vi "accelero_et_led.vi"() -> ()   [LabVIEW 2019]
uses:
  <vilib>/myRIO/Express VI/Onboard Devices/Accelerometer/Accelerometer Express VI.xnode
  <vilib>/myRIO/Instrument Drivers/Onboard Devices/Accelerometer/typedefs/Accelerometer Reference.ctl
  <vilib>/myRIO/Instrument Drivers/Onboard Devices/Accelerometer/Accelerometer.lvlib
  <vilib>/myRIO/Common/Instrument Driver Framework/myRIO v1.0/Accelerometer/typedefs/Accelerometer Channels List.ctl
  <vilib>/myRIO/Common/Instrument Driver Framework/myRIO v1.0/Accelerometer/typedefs/Accelerometer Channels Enum.ctl
  <vilib>/myRIO/Common/Instrument Driver Framework/Utilities/typedefs/myRIO Generic Hardware Reference.ctl
  <vilib>/myRIO/Common/Instrument Driver Framework/Utilities/typedefs/myRIO v1.0 Reference.ctl
  <vilib>/myRIO/Common/Instrument Driver Framework/Utilities/typedefs/Generic FPGA Reference.ctl
  <vilib>/myRIO/Common/Instrument Driver Framework/Utilities/typedefs/Hardware Version Enum.ctl
  <vilib>/myRIO/Instrument Drivers/Onboard Devices/Accelerometer/vis/Read.vi
  <vilib>/myRIO/Instrument Drivers/Onboard Devices/Accelerometer/vis/myRIO Accelerometer Open.xnode
  <vilib>/userDefined/High Color/nirio_resource_hc.ctl
  <vilib>/myRIO/Common/Instrument Driver Framework/Utilities/vis/Is FPGA Ref Available.vi
  <vilib>/myRIO/Common/Instrument Driver Framework/myRIO v1.0/DIO/typedefs/DIO Channels Enum.ctl
  <vilib>/myRIO/Common/Instrument Driver Framework/myRIO v1.0/DIO/typedefs/DIO Channels List.ctl
  <vilib>/myRIO/Instrument Drivers/Onboard IO/DIO/typedefs/DIO Reference.ctl
  <vilib>/myRIO/Instrument Drivers/Onboard IO/DIO/DIO.lvlib
  <vilib>/myRIO/Instrument Drivers/Onboard IO/DIO/vis/myRIO DIO Open.xnode
  <vilib>/myRIO/Common/Instrument Driver Framework/myRIO v1.0/DIO/vis/myRIO v1.1 Open DIO.vi
  <vilib>/myRIO/Express VI/Onboard IO/DI/DI Express VI.xnode
  <vilib>/myRIO/Instrument Drivers/Onboard IO/DIO/vis/Read.vi
  <vilib>/myRIO/Express VI/Onboard Devices/LED/LED Express VI.xnode
  <vilib>/myRIO/Instrument Drivers/Onboard IO/DIO/vis/Write.vi
  <vilib>/myRIO/Common/Instrument Driver Framework/myRIO v1.0/Accelerometer/vis/myRIO v1.1 Open Accelerometer.vi
panel:
  out "X 5":dbl(graph)
  out "X 4":dbl(graph)
  out "X 3":dbl(graph)
  out "X 2":dbl(graph)
  out "X":dbl(graph)
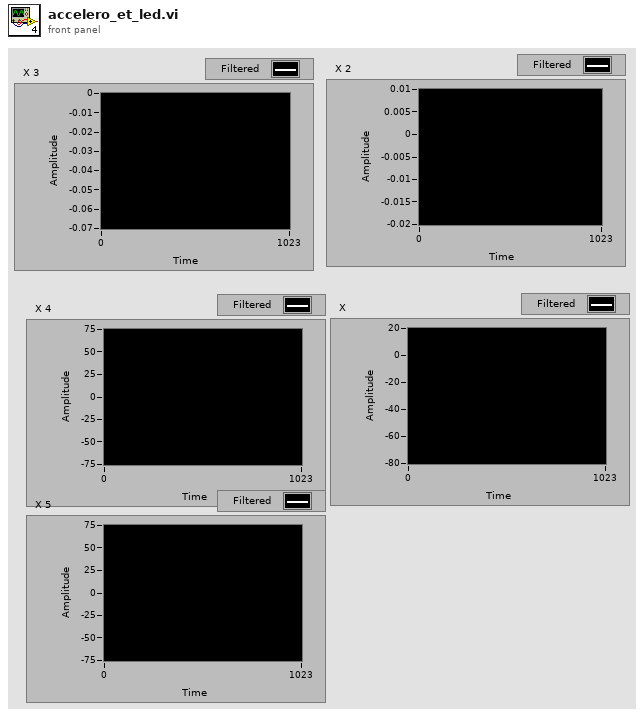
[diagram p1: front panel]
types:
  T1 = typedef "DIO.lvlib/DIO Reference.ctl" = cluster{"myRIO Reference":T2, "DIO Channels List":T6}
  T2 = typedef "myRIO Generic Hardware Reference.ctl" = cluster{"myRIO Model":T3, "myRIO Hardware Reference":T4}
  T3 = typedef "Hardware Version Enum.ctl" = enum16{"Unknown", "myRIO-1900", "myRIO-1950", "roboRIO", "NI ELVIS RIO CM", "ELVIS III"}
  T4 = typedef "myRIO v1.0 Reference.ctl" = cluster{"Generic FPGA Reference":T5, "Allow multiple opens":bool}
  T5 = typedef "Generic FPGA Reference.ctl" = refnum<k20>
  T6 = typedef "DIO Channels List.ctl" = T7[]
  T7 = typedef "DIO Channels Enum.ctl" = enum16{"Not Connected", "C/DIO0", "C/DIO1", "C/DIO2", "C/DIO3", "C/DIO4", "C/DIO5", "C/DIO6", "C/DIO7", "A/DIO0", "A/DIO1", "A/DIO2", "A/DIO3", "A/DIO4", "A/DIO5", "A/DIO6", "A/DIO7", "A/DIO8", "A/DIO9", "A/DIO10", "A/DIO11", "A/DIO12", "A/DIO13", "A/DIO14", "A/DIO15", "A/DIO16", "A/DIO17", "A/DIO18", "A/DIO19", "B/DIO0", "B/DIO1", "B/DIO2", "B/DIO3", "B/DIO4", "B/DIO5", "B/DIO6", "B/DIO7", "B/DIO8", "B/DIO9", "B/DIO10", "B/DIO11", "B/DIO12", "B/DIO13", "B/DIO14", "B/DIO15", "B/DIO16", "B/DIO17", "B/DIO18", "B/DIO19", "LED0", "LED1", "LED2", "LED3", "Button0", "DIO/DIO0", "DIO/DIO1", "DIO/DIO2", "DIO/DIO3", "DIO/DIO4", "DIO/DIO5", "DIO/DIO6", "DIO/DIO7", "DIO/DIO8", "DIO/DIO9", "SPI/CS0", "SPI/CS1", "SPI/CS2", "SPI/CS3", "LED RADIO (Green)", "LED RADIO (Red)", "LED COMM (Green)", "LED COMM (Red)", "LED MODE (Green)", "LED MODE (Red)"}
  T8 = typedef "nirio_resource_hc.ctl" = tag
  T9 = typedef "Accelerometer.lvlib/Accelerometer Reference.ctl" = cluster{"myRIO Reference":T2, "Accelerometer Channels List":T10, "LSB Weight":dbl}
  T10 = typedef "Accelerometer Channels List.ctl" = T11[]
  T11 = typedef "Accelerometer Channels Enum.ctl" = enum16{"Not Connected", "X-Axis", "Y-Axis", "Z-Axis"}
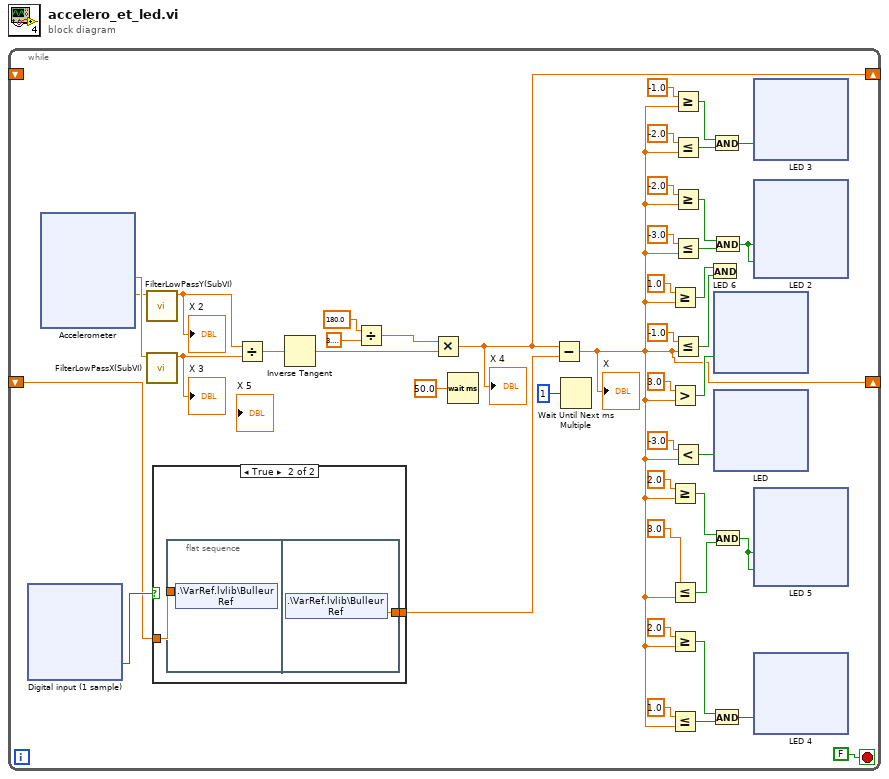
[diagram p0: block diagram]
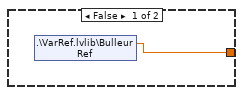
[diagram p2: hidden frame]
diagram:
  n1 = while {
    shift-right: [w5] -> _
    shift-left: _ -> [_]
    shift-right: [w4] -> _
    shift-left: _ -> [w2]
    stop <- FALSE stop-if-true
    n2 = xnode "Digital input (1 sample)"() -> ("A/DIO0 (Pin 11)"=w3:bool)  [unwired: 1 in, 1 out]
    n3 = xnode "Accelerometer"() -> ("X-Axis"=w9:dbl, "Y-Axis"=w8:dbl)  [unwired: 1 in, 2 out]
    n4 = call "FilterLowPassY(SubVI).vi"("Y-Axis"=w8) -> ("Filtered x"=w6:dbl)  [unwired: 9 in, 1 out]
    "X 2" <- w6
    n5 = call "FilterLowPassX(SubVI).vi"("X-Axis"=w9) -> ("Filtered x"=w7:dbl)  [unwired: 9 in, 1 out]
    "X 3" <- w7
    n6 = case shown="True" w3 {
      tunnel: w2 -> [_ w83]
      tunnel: [w81 w82] -> w1
      frame False {
        n7 = shared-variable ".\\VarRef.lvlib\\Bulleur Ref"() -> (w81:dbl)  [unwired: 1 in, 1 out]
      }
      frame True {
        n8 = flat-sequence {
          tunnel: w83 -> [w84]
          tunnel: [w85] -> w82
          frame #0 {
            n9 = shared-variable ".\\VarRef.lvlib\\Bulleur Ref"(w84) -> ()  [unwired: 1 in, 1 out]
          }
          frame #1 {
            n10 = shared-variable ".\\VarRef.lvlib\\Bulleur Ref"() -> (w85:dbl)  [unwired: 1 in, 1 out]
          }
        }
      }
    }
    n11 = Divide(x=w6, y=w7) -> (x/y=w44:dbl)
    n12 = Inverse Tangent(1:w44) -> (0:w43:dbl)
    n13 = Divide(x=180.0, y=3.141592653589793) -> (x/y=w40:dbl)
    n14 = Multiply(x=w40, y=w43) -> (x*y=w5:dbl)
    "X 4" <- w5
    n15 = Wait (ms)(milliseconds to wait=50.0) -> ()  [unwired: 1 out]
    n16 = Subtract(x=w5, y=w1) -> (x-y=w4:dbl)
    "X" <- w4
    n17 = Wait Until Next ms Multiple(millisecond multiple=1) -> ()  [unwired: 1 out]
    n18 = Greater Or Equal?(x=1.0, y=w4) -> (x >= y?=w27:bool)
    n19 = Greater?(x=3.0, y=w4) -> (0:w11:bool)
    n20 = Greater Or Equal?(x=2.0, y=w4) -> (x >= y?=w35:bool)
    n21 = Less Or Equal?(x=3.0, y=w4) -> (x <= y?=w33:bool)
    n22 = Greater Or Equal?(x=2.0, y=w4) -> (x >= y?=w31:bool)
    n23 = Less Or Equal?(x=1.0, y=w4) -> (x <= y?=w30:bool)
    n24 = Greater Or Equal?(x=-1.0, y=w4) -> (x >= y?=w23:bool)
    n25 = Less Or Equal?(x=-2.0, y=w4) -> (x <= y?=w22:bool)
    n26 = Greater Or Equal?(x=-2.0, y=w4) -> (x >= y?=w19:bool)
    n27 = Less Or Equal?(x=-3.0, y=w4) -> (x <= y?=w17:bool)
    n28 = Less Or Equal?(x=-1.0, y=w4) -> (x <= y?=w26:bool)
    n29 = Less?(x=-3.0, y=w4) -> (x < y?=w16:bool)
    n30 = And(x=w27, y=w26) -> ()  [unwired: 1 out]
    n31 = And(x=w23, y=w22) -> (x .and. y?=w14:bool)
    n32 = And(x=w31, y=w30) -> (x .and. y?=w13:bool)
    n33 = And(x=w19, y=w17) -> (x .and. y?=w15:bool)
    n34 = And(x=w35, y=w33) -> (x .and. y?=w12:bool)
    n35 = xnode "LED 6"("LED3"=w11) -> ()  [unwired: 1 in, 1 out]
    n36 = xnode "LED"("LED0"=w16) -> ()  [unwired: 1 in, 1 out]
    n37 = xnode "LED 3"("LED1"=w14) -> ()  [unwired: 1 in, 1 out]
    n38 = xnode "LED 2"("LED0"=w15, "LED1"=w15) -> ()  [unwired: 1 in, 1 out]
    n39 = xnode "LED 5"("LED2"=w12, "LED3"=w12) -> ()  [unwired: 1 in, 1 out]
    n40 = xnode "LED 4"("LED2"=w13) -> ()  [unwired: 1 in, 1 out]
  }
